vi "get_wavelength_wavenumber.vi"(8 "error in":errorcluster, 10 "Measure Type":enum16{"Wavelength", "Wavenumber"}(ring), 11 "address":string) -> (0 "error out":errorcluster, 3 "Wavelength/Wavenuumber":dbl)   [LabVIEW 2020]
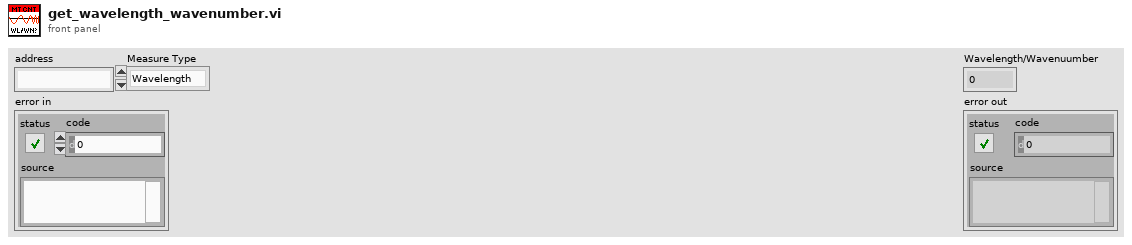
[diagram p1: front panel]
types:
  T1 = enum16{"Standard", "Buffered", "CRLF", "Immediate"}
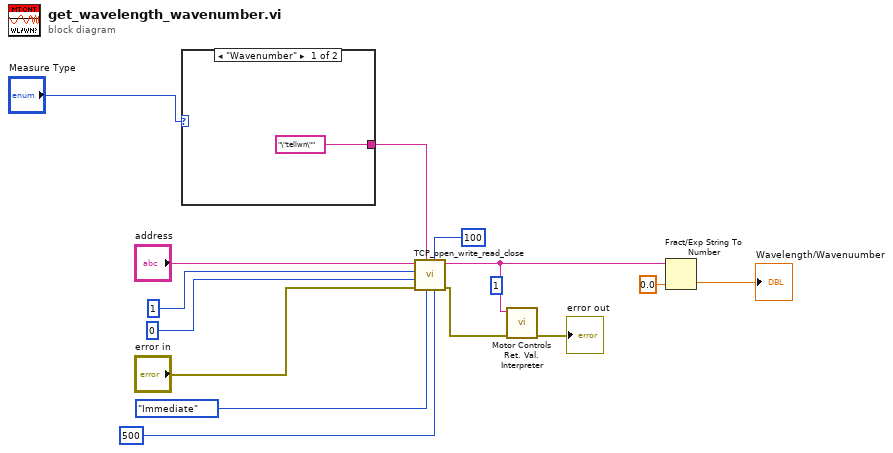
[diagram p0: block diagram]
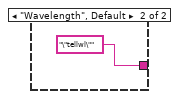
[diagram p2: hidden frame]
diagram:
  (unwired) 1 ("default (0 I32)")
  n1 = case shown="\"Wavenumber\"" "Measure Type" {
    tunnel: ["\"tellwn\"" "\"tellwl\""] -> w5
    frame "Wavenumber" {
    }
    frame "Wavelength", Default {
    }
  }
  n2 = call "TCP_open_write_read_close.vi"("timeout ms (25000)"=500, "bytes to read"=100, "mode (standard)"=T1."Immediate", "write string"=w5, "error in"="error in", "local port (0)"=u16 0, "remote port or service name"=u16 1, "address"="address") -> ("error out"=w8:errorcluster, "read string"=w3:string)  [unwired: 2 in]
  n3 = call "Motor Controls Ret. Val. Interpreter.vi"("error in"=w8, "Command Return"=w3) -> ("error out"=→"error out":errorcluster)  [unwired: 8 in, 1 out]
  n4 = Fract/Exp String To Number(string=w3, default (0 dbl)=0.0 ("default (0 DBL)")) -> (number=→"Wavelength/Wavenuumber":dbl)  [unwired: 2 in, 1 out]
